vi "fifo_cam_laser_comp.vi"() -> ()   [LabVIEW 2019]
uses:
  <vilib>/rvi/Emulation/niFpgaGetClockAttributes.vi
  <vilib>/rvi/Emulation/niFpgaSctlEmulationGetInTimedLoop.vi
  <vilib>/rvi/Emulation/niFpgaEmulationReportErrorSimple.vi
  <vilib>/rvi/Emulation/niFpgaProcessEmulError.vi
  <vilib>/rvi/eio/common/nirviEmuTemplateMethod_errors.vi
  <vilib>/rvi/Emulation/niFpgaCriticalErrorInLSC.vi
  <vilib>/rvi/DataTransferAndStorage/Container/Common/niFpgaContainerExecOnDevCompGetState.vi
  <vilib>/rvi/Emulation/niFpgaEmulationIsFPGAContextNoSignature.vi
  <vilib>/rvi/errors/niFpgaSetErrorForExecOnDevCompSimple.vi
  <vilib>/rvi/eio/common/nirviEmuReportErrorAndStop.vi
  <vilib>/rvi/DataTransferAndStorage/Container/Common/niFpgaContainerGetUniqueNameForEmu.vi
  <vilib>/rvi/FIFO/Fifo_Resource/nirvififoEmulationSetSize.vi
  <vilib>/rvi/FIFO/Fifo_Resource/nirviFifoEmulationQueueMgr.vi
  <instcachedir>/0/nirviFifoEmulationQueueMgr_E5CAEC123FF24DC58D834DCA3CDAA9B5.lvgen/nirviFifoEmulationQueueMgr_E5CAEC123FF24DC58D834DCA3CDAA9B5_001.vi
  <vilib>/rvi/FIFO/Fifo_Resource/nirvififoEmulationDetermineInputValidOut.vi
  <vilib>/rvi/FIFO/Fifo_Resource/nirvififoEmulationCreateLock.vi
  <vilib>/rvi/FIFO/Fifo_Resource/nirvififoEmulationObtainLock.vi
  <vilib>/rvi/FIFO/Fifo_Resource/nirvififoEmulationReleaseLock.vi
  <vilib>/rvi/occurrence/nirviWaitOnOccurrenceBase.vi
  <vilib>/rvi/errors/nirviReportUnexpectedCaseInternalError.vi
  <vilib>/rvi/errors/nirviReportUnexpectedCaseInternalError (U32).vi
  <vilib>/Utility/error.llb/Clear Errors.vi
  <vilib>/rvi/interface/RandomDataEmulation/niFpgaRandomDataHandleErrors.vi
  <instcachedir>/0/nirviFifoEmulationQueueMgr_E5CAEC123FF24DC58D834DCA3CDAA9B5.lvgen/nirviFifoEmulationQueueMgr_E5CAEC123FF24DC58D834DCA3CDAA9B5_000.vi
  <vilib>/eio/EIONode/EIONode.xnode
  <vilib>/rvi/DataTransferAndStorage/Container/XNode/niFpgaContainer.xnode
  <vilib>/rvi/FIFO/Fifo_Resource/niFpgaFifoEmulationRefIn.vi
panel:
  in  "Timeout":i32=-1
  in  "Cam":bool
  out "cam report":bool
  in  "stop":bool
  out "volt":i16
  out "Count":u32 caption="Tick Count(uSec)"
  out "Load":u16
  in  "Count(uSec)":u32
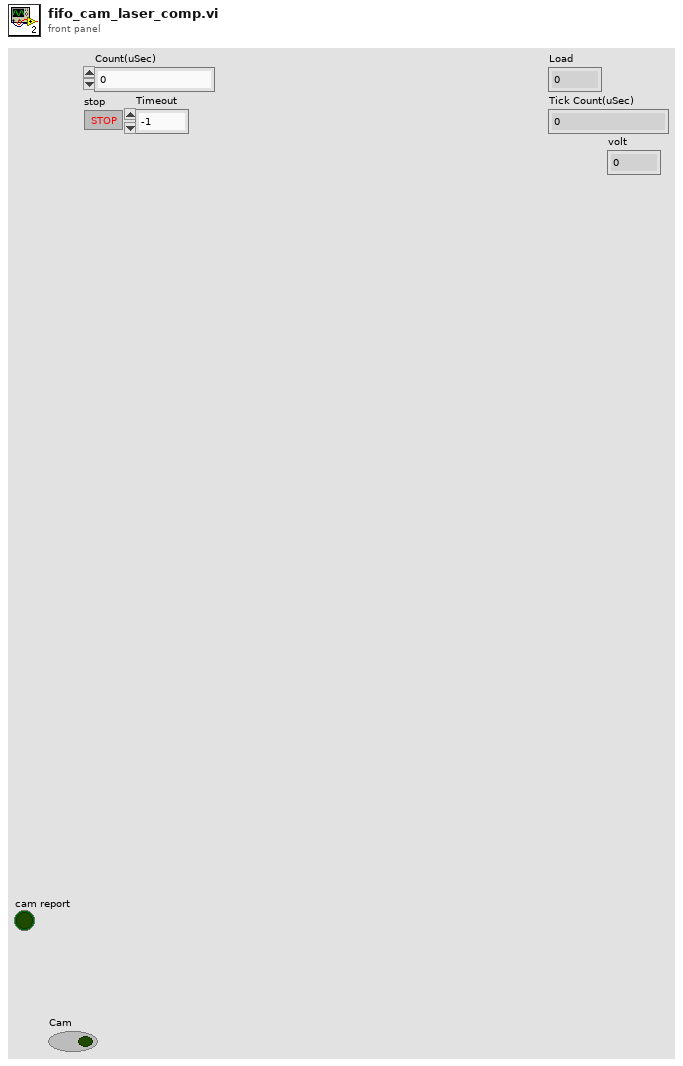
[diagram p1: front panel]
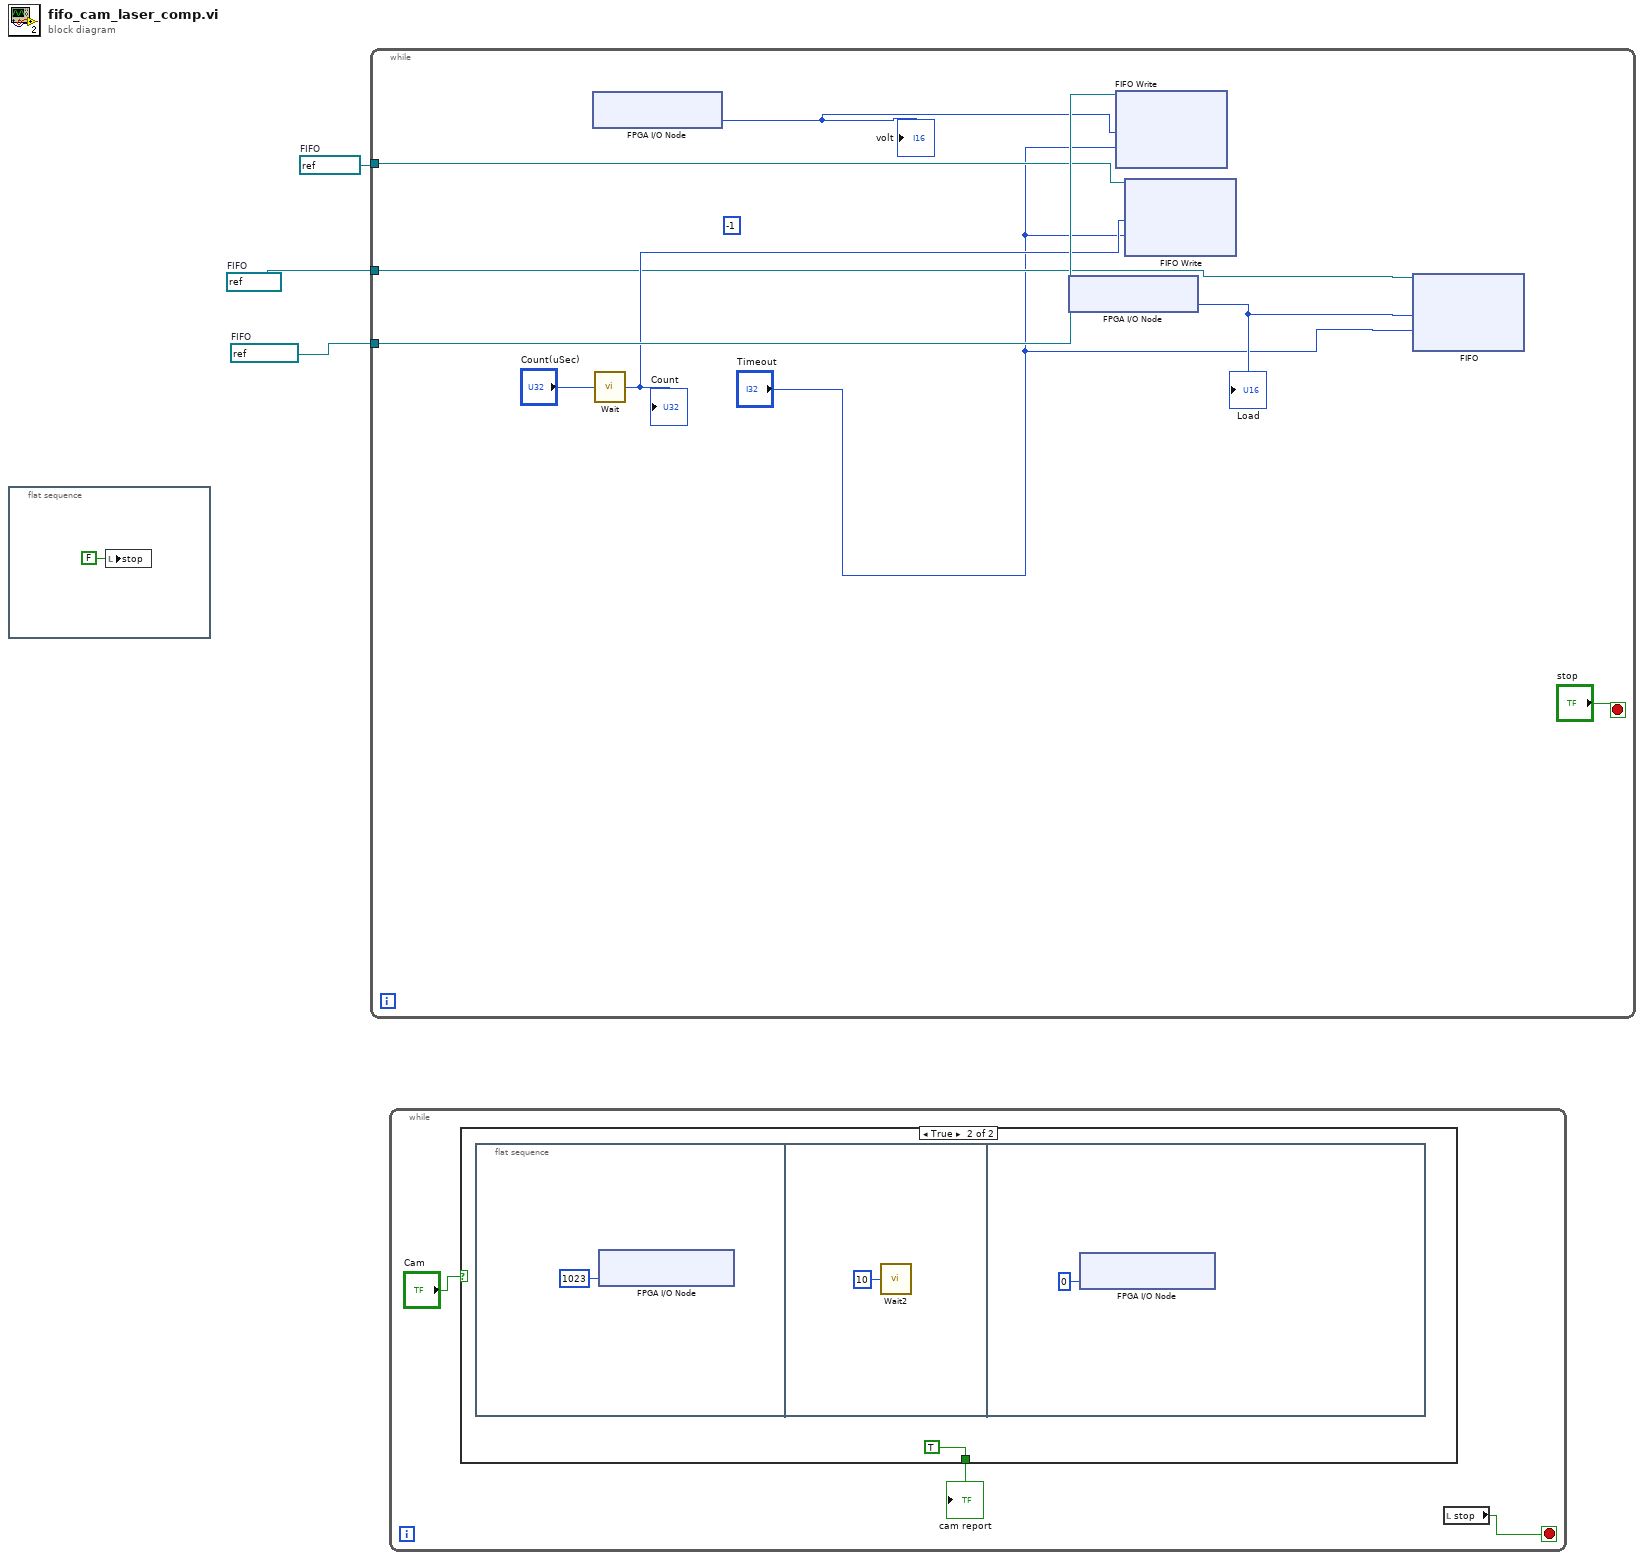
[diagram p0: block diagram]
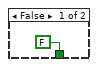
[diagram p2: hidden frame]
diagram:
  w1 = refnum<k21> "Laser"  # FIFO
  w2 = refnum<k21> "Count"  # FIFO
  w3 = refnum<k21> "Voltage"  # FIFO
  n1 = flat-sequence {
    frame #0 {
      n2 = local write "stop"(FALSE ("stop")) -> ()
    }
  }
  n3 = while {
    tunnel: w3 -> [w11]
    tunnel: w2 -> [w9]
    tunnel: w1 -> [w7]
    stop <- "stop" stop-if-true
    (unwired) -1
    n4 = xnode "FPGA I/O Node"() -> ("ConnectorC/AI0"=w10:i16)  [unwired: 1 in, 1 out]
    "volt" <- w10
    n5 = call "Wait"("Count(uSec)"="Count(uSec)") -> ("Tick Count(uSec)"=w8:u32)
    "Count" <- w8
    n6 = xnode "FPGA I/O Node"() -> ("ConnectorA/AI1"=w6:u16)  [unwired: 1 in, 1 out]
    "Load" <- w6
    n7 = xnode ("FIFO Write")("Element"=w10, "Timeout"="Timeout", "FIFO In"=w11) -> ()  [unwired: 2 out]
    n8 = xnode ("FIFO Write")("Element"=w8, "Timeout"="Timeout", "FIFO In"=w9) -> ()  [unwired: 2 out]
    n9 = xnode "FIFO"("Element"=w6, "Timeout"="Timeout", "FIFO In"=w7) -> ()  [unwired: 2 out]
  }
  n10 = while {
    stop <- w15 stop-if-true
    n11 = case shown="True" "Cam" {
      tunnel: [FALSE TRUE] -> w14
      frame False {
      }
      frame True {
        n12 = flat-sequence {
          frame #0 {
            n13 = xnode "FPGA I/O Node"("ConnectorC/AO0"=i16 1023) -> ()  [unwired: 1 in, 1 out]
          }
          frame #1 {
            n14 = call "Wait2"("Count(mSec)"=u32 10) -> ()  [unwired: 1 out]
          }
          frame #2 {
            n15 = xnode "FPGA I/O Node"("ConnectorC/AO0"=i16 0) -> ()  [unwired: 1 in, 1 out]
          }
        }
      }
    }
    "cam report" <- w14
    n16 = local read "stop"() -> (w15:bool)
  }
